vi "Remove.vi"() -> ()   [LabVIEW 2024, in "TypedCircularBuffer.Tests.Units.lvlib"]
uses:
  TypedCircularBuffer.Tests.Units.lvlib
  <vilib>/addons/_JKI Toolkits/Caraya/classes/Assert/Assert.lvclass
  <vilib>/addons/_JKI Toolkits/Caraya/classes/Test/Test.lvclass
  TypedCircularBuffer.lvclass
  <vilib>/addons/_JKI Toolkits/Caraya/classes/Assert/Assert True.vi
  <vilib>/addons/_JKI Toolkits/Caraya/classes/Assert/Assert False.vi
  Type.ctl
panel:
  out "element":T1
  in  "expected":i32[](array[numeric])=[2, 3, 4, 5, 6, 7, 8, 9, 10]
  out "Flushed Buffer":T1[](array[typedef])
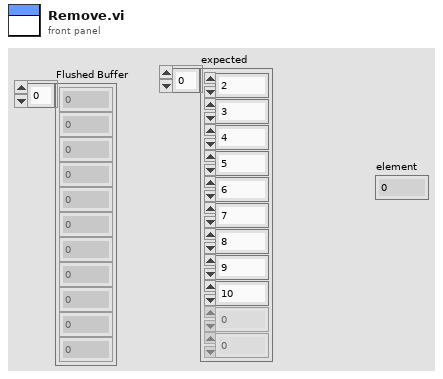
[diagram p1: front panel]
types:
  T1 = typedef "TypedCircularBuffer.lvclass/Type.ctl" = i32
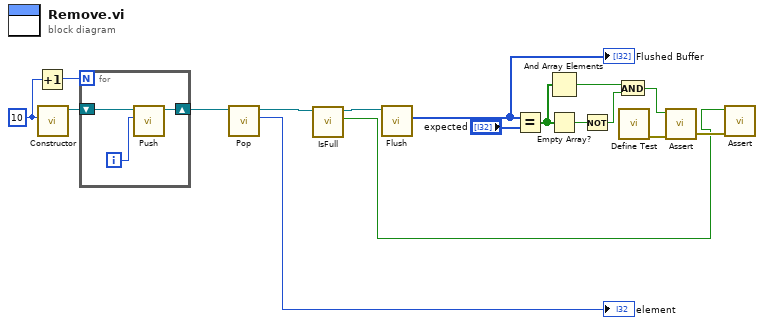
[diagram p0: block diagram]
diagram:
  w15 = u32 10 ("Capacity")
  n1 = Increment(x=w15) -> (x+1=w16:u32)
  n2 = call "Constructor.vi"("Capacity"=w15) -> ("TypedCircularBuffer out"=w17:refnum<class "TypedCircularBuffer.lvclass">)  [unwired: 10 in]
  n3 = for {
    N: w16 -> [_]
    shift-right: [w19] -> w6
    shift-left: w17 -> [w20]
    i -> [w18]
    n4 = call "Push.vi"("Element"=w18, "TypedCircularBuffer in"=w20) -> ("TypedCircularBuffer out"=w19:refnum<class "TypedCircularBuffer.lvclass">)  [unwired: 7 in, 2 out]
  }
  n5 = call "Pop.vi"("TypedCircularBuffer in"=w6) -> ("element"=→"element":T1, "TypedCircularBuffer out"=w4:refnum<class "TypedCircularBuffer.lvclass">)  [unwired: 8 in, 1 out]
  n6 = call "IsFull.vi"("TypedCircularBuffer in"=w4) -> ("Full?"=w1:bool, "TypedCircularBuffer out"=w3:refnum<class "TypedCircularBuffer.lvclass">)  [unwired: 9 in]
  n7 = call "Flush.vi"("TypedCircularBuffer in"=w3) -> ("Flushed Buffer"=w8:T1[])  [unwired: 9 in, 1 out]
  "Flushed Buffer" <- w8
  n8 = Equal?(x=w8, y="expected") -> (x = y?=w11:bool[])
  n9 = And Array Elements(Boolean array=w11) -> (logical AND=w14:bool)
  n10 = Empty Array?(array=w11) -> (empty?=w13:bool)
  n11 = Not(x=w13) -> (.not. x?=w12:bool)
  n12 = And(x=w14, y=w12) -> (x .and. y?=w10:bool)
  n13 = call <vilib>:"Define Test.vi"() -> ("error out"=w9:errorcluster)  [unwired: 10 in, 1 out]
  n14 = call-poly <vilib>:"Assert.vi"("error in (no error)"=w9, "True?"=w10) -> ("error out"=w2:errorcluster)  [unwired: 8 in, 1 out]
  n15 = call-poly <vilib>:"Assert.vi"("error in (no error)"=w2, "False?"=w1) -> ()  [unwired: 8 in, 2 out]
